vi "Get ContentRectBounds.vi"(8 "错误输入":errorcluster, 11 "Mlistbox Ref":refnum<vi>) -> (0 "错误输出":errorcluster, 2 "ContentRectBounds":T1, 3 "Mlistbox Ref Dup":refnum<vi>)   [LabVIEW 2012, in "Mlistbox Tools.lvlib"]
uses:
  Mlistbox Tools.lvlib
  <vilib>/Utility/miscctls.llb/LVBoundsTypeDef.ctl
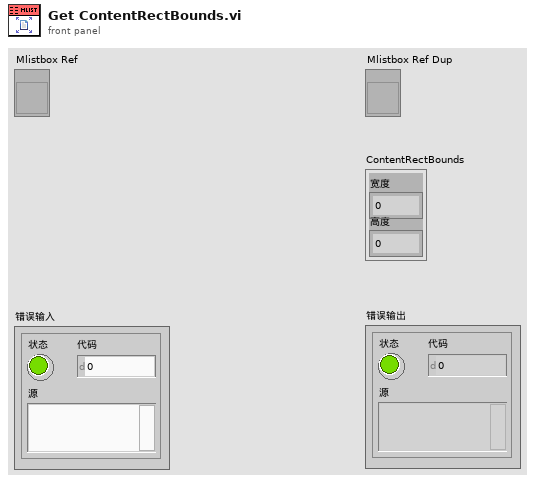
[diagram p1: front panel]
types:
  T1 = typedef "LVBoundsTypeDef.ctl" = cluster{"Width":u32, "Height":u32}
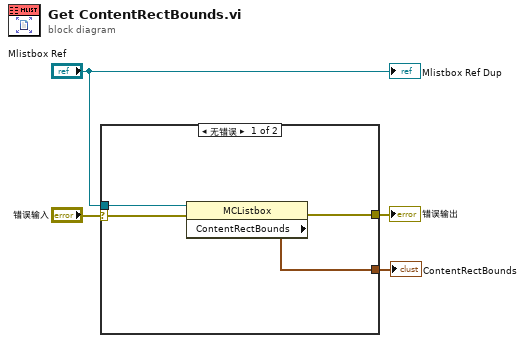
[diagram p0: block diagram]
diagram:
  n1 = case shown="无错误" "错误输入" {
    selector: "错误输入" -> [w7 w9]
    tunnel: [w5 w9] -> w3
    tunnel: "Mlistbox Ref" -> [w8 _]
    tunnel: [w6 _] -> w1
    frame No Error {
      n2 = property class="MCListbox"(reference=w8, error in=w7) -> (error out=w5:errorcluster, "ContentRectBounds"=w6:T1)  [unwired: 1 out]
    }
    frame Error {
    }
  }
  "错误输出" <- w3
  "ContentRectBounds" <- w1
  "Mlistbox Ref Dup" <- "Mlistbox Ref"
